vi "ReadWriteTablesTest_1212_K7.vi"() -> ()   [LabVIEW 2018]
uses:
  <vilib>/Platform/TimedLoop/XDataNode/XDataNode.xnode
  <vilib>/Platform/TimedLoop/XDataNode/nitl_modes.ctl
  <vilib>/Platform/TimedLoop/XDataNode/XDNodeRunTimeDep.lvlib
  <vilib>/Platform/TimedLoop/XDataNode/wakeup.ctl
  <vilib>/Platform/TimedLoop/XDataNode/timing_clust.ctl
  <vilib>/rvi/DataTransferAndStorage/Container/XNode/niFpgaContainer.xnode
  <vilib>/eio/EIONode/EIONode.xnode
  <vilib>/rvi/Memory/Memory_Emulation/nirvimemoryEmulation.vi
  <vilib>/rvi/eio/common/nirviEmuTemplateMethod_errors.vi
  <vilib>/rvi/Memory/Memory_Emulation/nirvimemoryFastEmulation.vi
  Program_Files/Labview2018/MAIN/instr.lib/_niInstr/Basic Elements/v1/FPGA/niInstr Basic Elements v1 FPGA.lvlib
  GeneratorStates.ctl
panel:
  out "pulse period":u32
  in  "TrigDigi":bool
  in  "Vi_Trig/nStage_Trig":bool=TRUE
  in  "Trig In":bool
  out "IO Module\\trig_in Edge Detected":bool=TRUE
  in  "Delay bw waves [cycles]":u32
  in  "Waves Per Pixel":i16=1
  out "busy_ni2c":bool
  in  "Trig Selection":bool
  in  "Trig Reset":bool
  in  "Offset_CH1":u32
  in  "Offset_CH0":u32
  in  "START_CH":bool
  in  "Clock SEL":bool
  out "ReadDataI2c":fxp<+,8,8>
  in  "StartRDI2c":bool
  in  "StartWRI2c":bool
  in  "DataI2c5":fxp<+,8,8>
  in  "DataI2c4":fxp<+,8,8>
  in  "DataI2c3":fxp<+,8,8>
  in  "DataI2c2":fxp<+,8,8>
  in  "DataI2c1":fxp<+,8,8>
  in  "DataI2c0":fxp<+,8,8>
  out "START MAST CH1":bool
  out "START MAST CH0":bool
  in  "WRITE MEM CH1":bool
  in  "DDS/ARB CH1":bool=TRUE
  in  "LastAddress_CH1":u32
  in  "Increment_CH1":u32=8
  in  "EN_CH1":bool
  in  "ClkEnable":bool
  in  "WriteAddress":u32
  in  "WriteData":fxp<+,14,14>
  in  "WRITE MEM CH0":bool
  out "Data16":fxp<+,14,14>=8192.0
  in  "StopAddress8_CH1":u32=6143
  out "Data15":fxp<+,14,14>=8192.0
  in  "StopAddress7_CH1":u32=6142
  out "Data14":fxp<+,14,14>=8192.0
  in  "StopAddress6_CH1":u32=6141
  out "Data13":fxp<+,14,14>=8192.0
  in  "StopAddress5_CH1":u32=6140
  out "Data12":fxp<+,14,14>=8192.0
  in  "StopAddress4_CH1":u32=6139
  out "Data11":fxp<+,14,14>=8192.0
  in  "StopAddress3_CH1":u32=6138
  out "Data10":fxp<+,14,14>=8192.0
  in  "StopAddress2_CH1":u32=6137
  out "Data9":fxp<+,14,14>=8192.0
  in  "StopAddress1_CH1":u32=6136
  out "Data8":fxp<+,14,14>=8192.0
  in  "StopAddress8_CH0":u32=6143
  out "Data7":fxp<+,14,14>=8192.0
  in  "StopAddress7_CH0":u32=6142
  out "Data6":fxp<+,14,14>=8192.0
  in  "StopAddress6_CH0":u32=6141
  out "Data5":fxp<+,14,14>=8192.0
  in  "StopAddress5_CH0":u32=6140
  out "Data4":fxp<+,14,14>=8192.0
  in  "StopAddress4_CH0":u32=6139
  out "Data3":fxp<+,14,14>=8192.0
  in  "StopAddress3_CH0":u32=6138
  out "Data1":fxp<+,14,14>=8192.0
  in  "StopAddress1_CH0":u32=6136
  in  "StopAddress2_CH0":u32=6137
  in  "LastAddress_CH0":u32
  out "Data2":fxp<+,14,14>=8192.0
  in  "EN_CH0":bool
  in  "StartAddress7_CH1":u32=6
  in  "StartAddress4_CH1":u32=3
  in  "StartAddress1_CH1":u32
  in  "StartAddress8_CH1":u32=7
  in  "StartAddress6_CH1":u32=5
  in  "StartAddress5_CH1":u32=4
  in  "StartAddress2_CH1":u32=1
  in  "StartAddress3_CH1":u32=2
  in  "StartAddress8_CH0":u32=7
  in  "StartAddress7_CH0":u32=6
  in  "StartAddress6_CH0":u32=5
  in  "StartAddress5_CH0":u32=4
  in  "StartAddress4_CH0":u32=3
  in  "StartAddress3_CH0":u32=2
  in  "StartAddress2_CH0":u32=1
  in  "StartAddress1_CH0":u32
  in  "SysReset":bool
  in  "IO Module\\trig_out":bool
  out "IO Module\\lockedfast":bool
  out "IO Module\\trig_in":bool=TRUE
  in  "DDS/ARB CH0":bool=TRUE
  in  "Increment_CH0":u32=8
  out "error out":errorcluster
  in  "error in (no error)":errorcluster
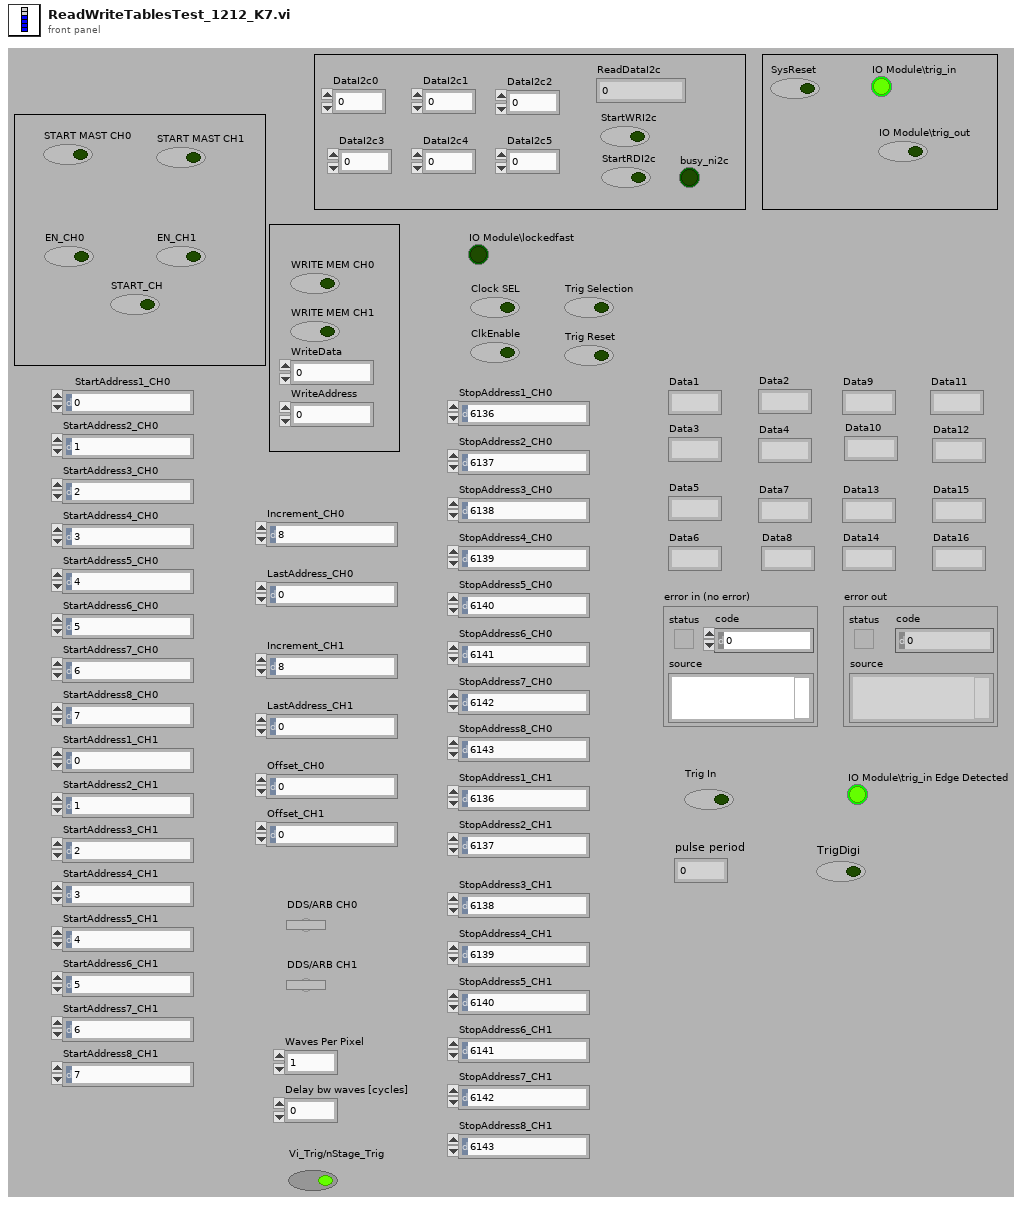
[diagram p1: front panel]
types:
  T1 = typedef "GeneratorStates.ctl" = enum16{"Wait For Trigger", "Wait For Pulse", "Check Pulse Count", "Delay"}
  T2 = typedef "XDNodeRunTimeDep.lvlib/timing_clust.ctl" = cluster{"Expected End [f-1]":u64, "Actual End [f-1]":u64, "Finished Late? [f-1]":bool, "Expected End [i-1]":u64, "Actual End [i-1]":u64, "Finished Late? [i-1]":bool, "Expected Start [i]":u64, "Actual Start [i]":u64, "Expected Start [f]":u64, "Actual Start [f]":u64, "Source Name":string, "Structure Name":string, "Period":i64, "Deadline":i64, "Offset":i64, "Start":i64, "Priority":i32, "Timeout":i32, "Mode":T3, "Wakeup Reason":T4, "Error":errorcluster, "Source Type":string, "Secondary Source Type":string, "Global End Time":u64, "Global Start Time":u64, "Frame Duration":u64, "Iteration Duration":u64, "Assigned CPU":i32, "I/O Scan Engine Mode":u32}
  T3 = typedef "XDNodeRunTimeDep.lvlib/nitl_modes.ctl" = enum32{"No Change", "Process missed periods, maintain original phase", "Discard missed periods, maintain original phase", "Process missed periods, ignore original phase", "Discard missed periods, ignore original phase"}
  T4 = typedef "XDNodeRunTimeDep.lvlib/wakeup.ctl" = enum32{"Normal", "Aborted", "Asynchronous wakeup", "Timing source error", "Timed loop error", "Timeout"}
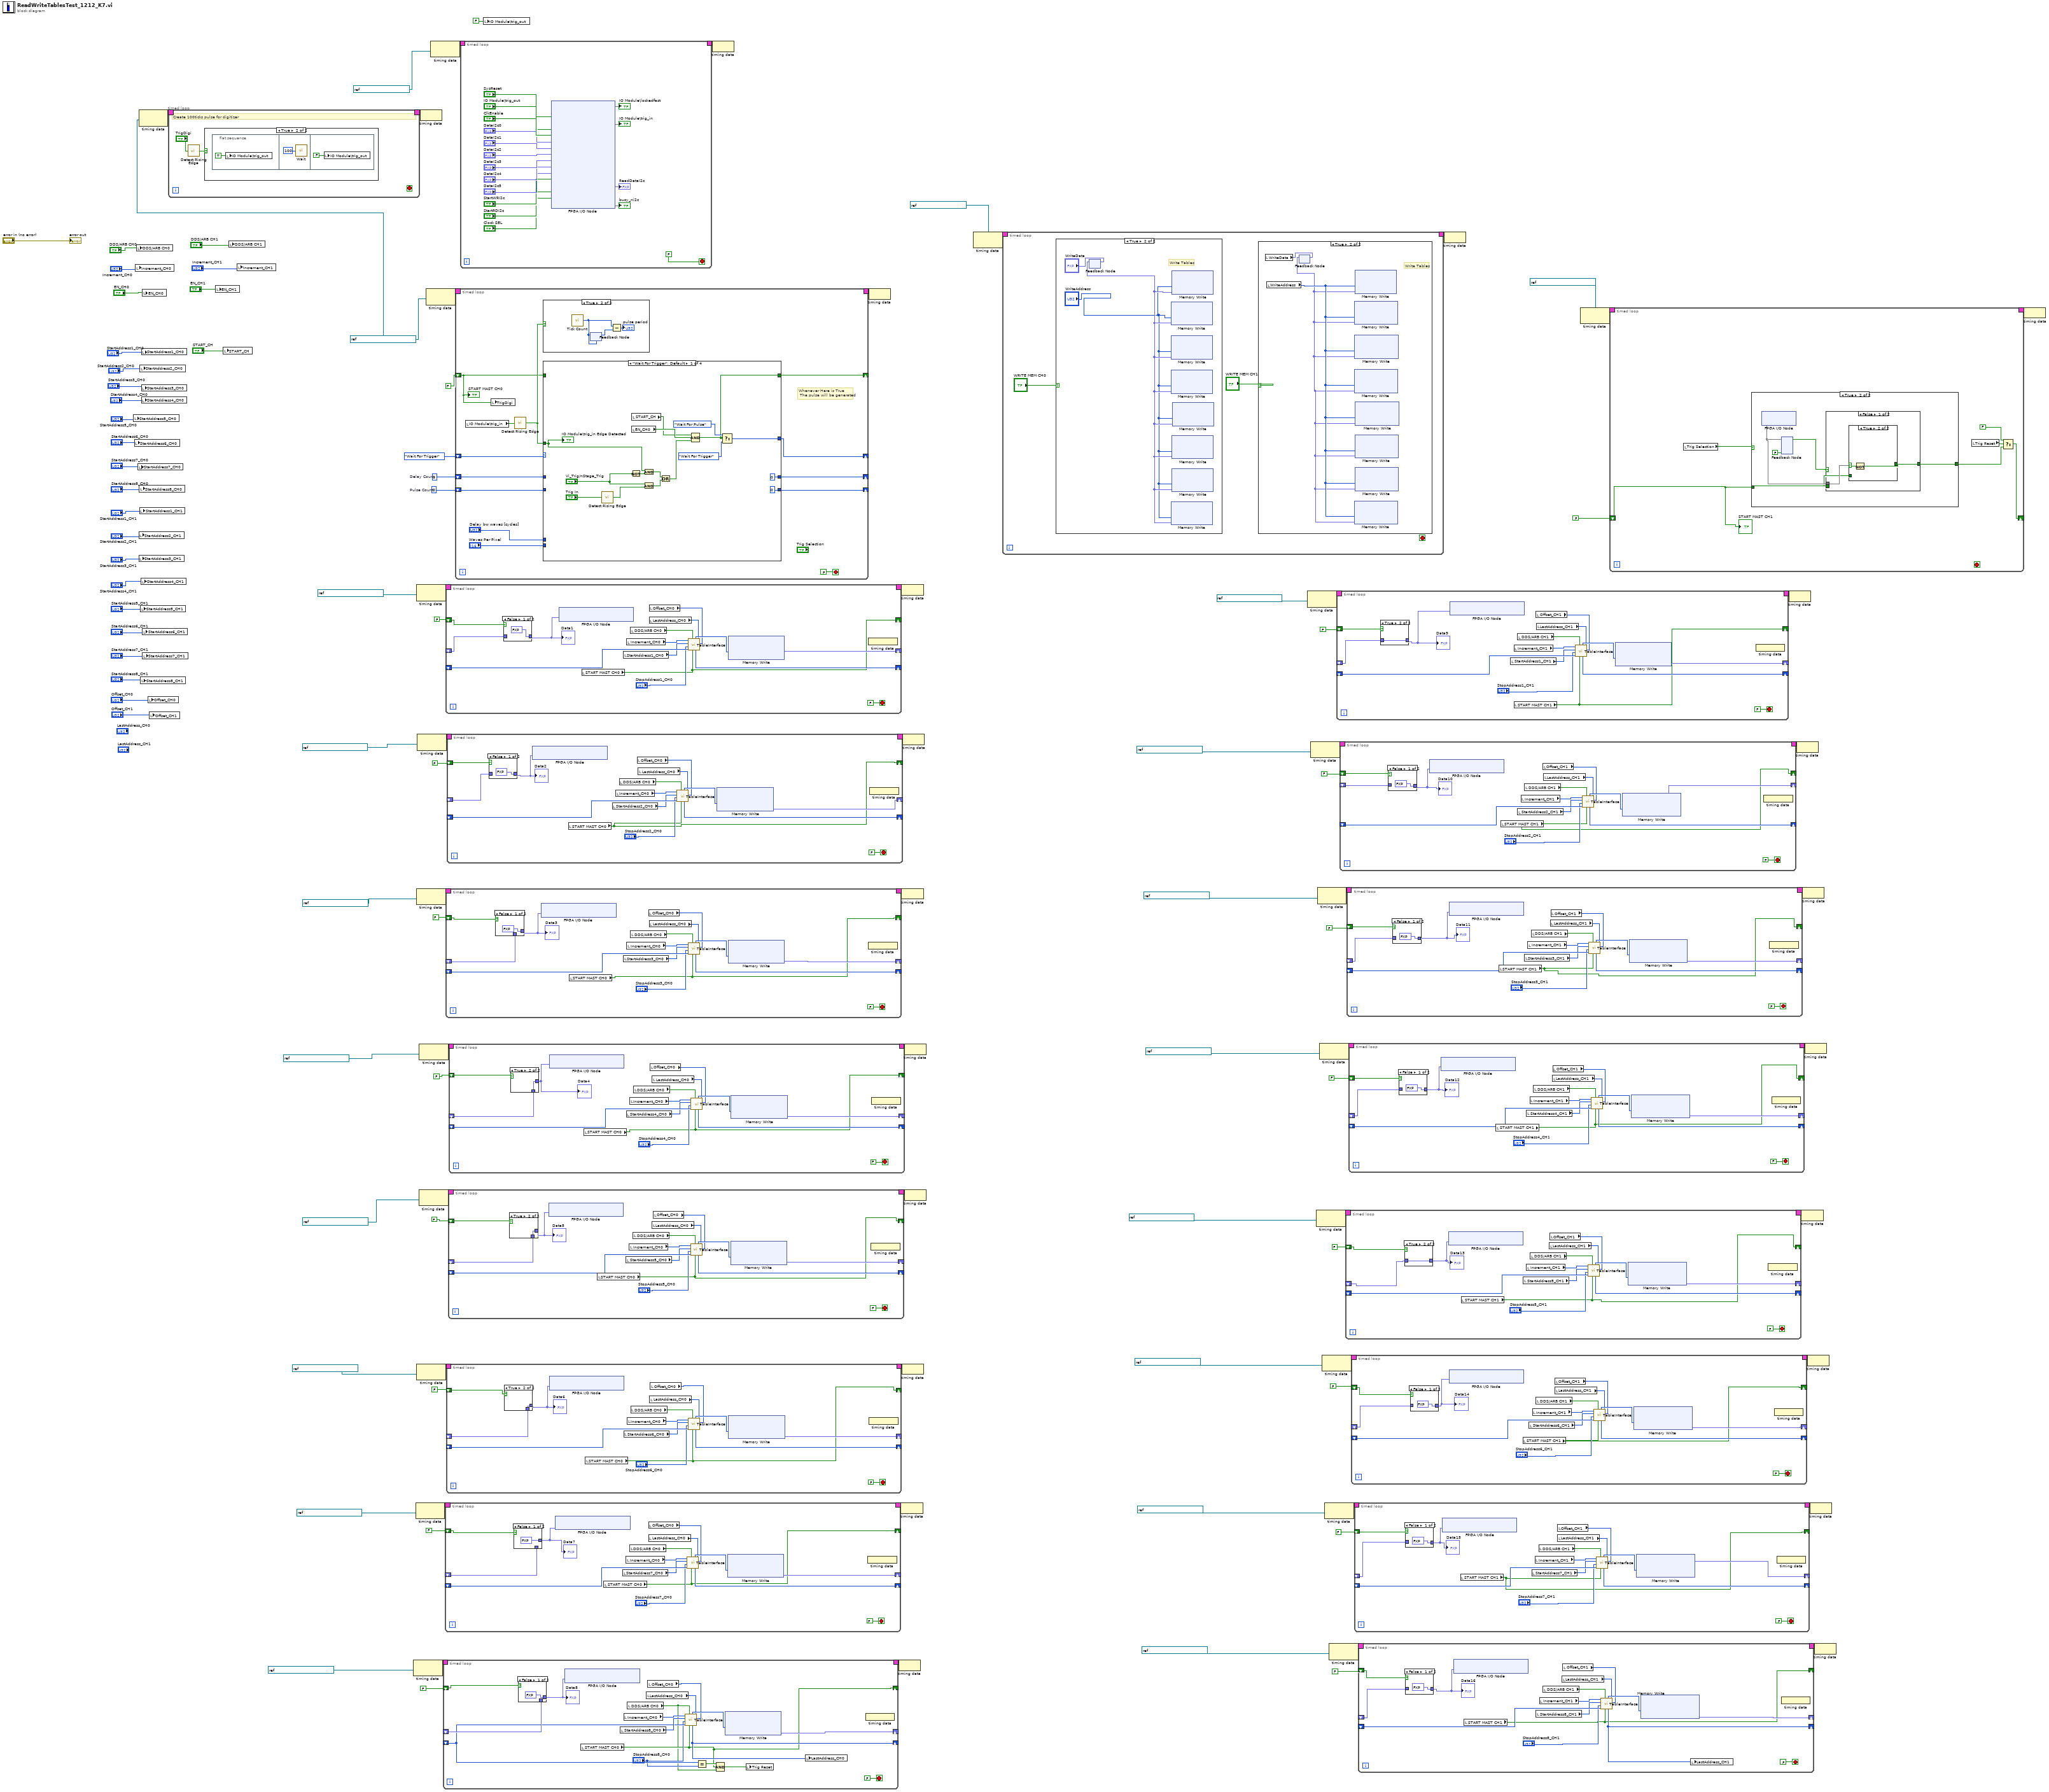
[diagram p0: block diagram]
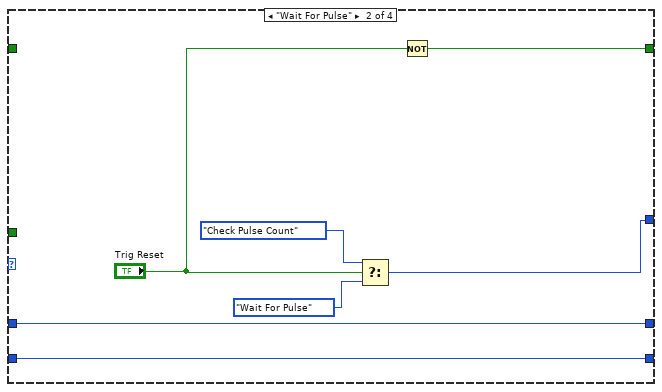
[diagram p4: hidden frame]
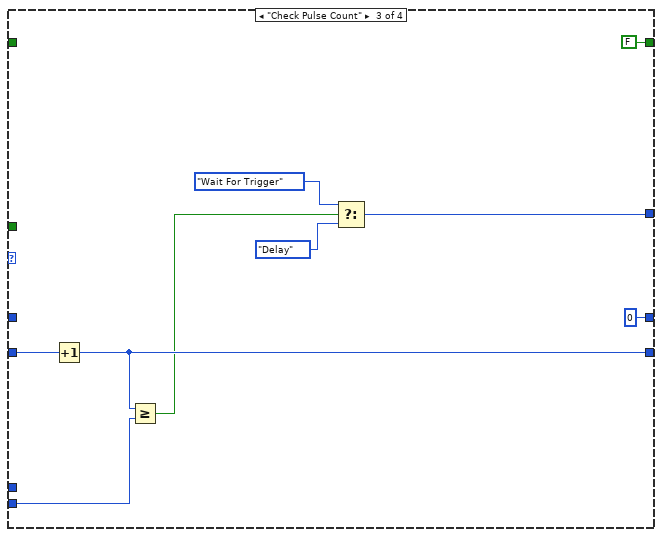
[diagram p5: hidden frame]
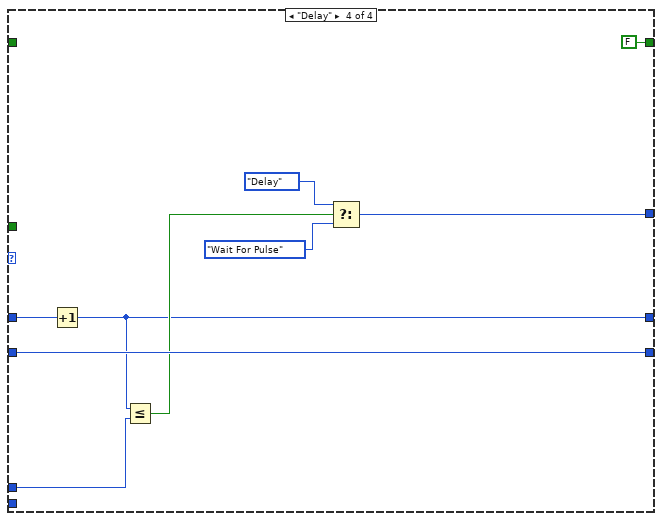
[diagram p6: hidden frame]
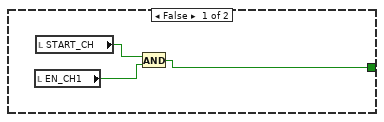
[diagram p7: hidden frame]
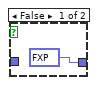
[diagram p15: hidden frame]
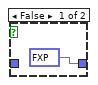
[diagram p19: hidden frame]
diagram:
  w6 = u32 0  # Delay Count
  w7 = i16 0  # Pulse Count
  w2 = refnum<k21> "IO Module\\iomodclipclock0" ("Source Name")
  n1 = local write "StartAddress5_CH0"("StartAddress5_CH0") -> ()
  n2 = local write "StartAddress6_CH0"("StartAddress6_CH0") -> ()
  n3 = local write "Increment_CH0"("Increment_CH0") -> ()
  n4 = local write "DDS/ARB CH0"("DDS/ARB CH0") -> ()
  n5 = local write "StartAddress7_CH0"("StartAddress7_CH0") -> ()
  n6 = node-c288(w2) -> (w4:T2)
  n7 = local write "StartAddress2_CH1"("StartAddress2_CH1") -> ()
  n8 = local write "StartAddress3_CH1"("StartAddress3_CH1") -> ()
  n9 = local write "StartAddress8_CH0"("StartAddress8_CH0") -> ()
  n10 = local write "StartAddress1_CH1"("StartAddress1_CH1") -> ()
  n11 = local write "StartAddress2_CH0"("StartAddress2_CH0") -> ()
  n12 = local write "StartAddress5_CH1"("StartAddress5_CH1") -> ()
  n13 = local write "StartAddress8_CH1"("StartAddress8_CH1") -> ()
  n14 = local write "StartAddress4_CH1"("StartAddress4_CH1") -> ()
  n15 = local write "StartAddress1_CH0"("StartAddress1_CH0") -> ()
  n16 = local write "StartAddress3_CH0"("StartAddress3_CH0") -> ()
  n17 = local write "StartAddress4_CH0"("StartAddress4_CH0") -> ()
  n18 = local write "EN_CH0"("EN_CH0") -> ()
  n19 = local write "StartAddress6_CH1"("StartAddress6_CH1") -> ()
  n20 = local write "StartAddress7_CH1"("StartAddress7_CH1") -> ()
  n21 = local write "Offset_CH0"("Offset_CH0") -> ()
  n22 = local write "Offset_CH1"("Offset_CH1") -> ()
  n23 = timed-loop {
    timing: w4 -> [_]
    timing-out: [_] -> w3
    stop <- _ stop-if-true
    # "Create 100ticks pulse for digitizer"
    n24 = call "Detect Rising Edge.vi"("signal"="TrigDigi") -> ("edge detected"=w111:bool)  [unwired: 14 in]
    n25 = case shown="True" w111 {
      frame False {
      }
      frame True {
        n26 = flat-sequence {
          frame #0 {
            n27 = local write "IO Module\\trig_out"(TRUE ("IO Module\\trig_out")) -> ()
          }
          frame #1 {
            n28 = call "Wait"("Count(Ticks)"=u32 100 ("Count(uSec)")) -> ()  [unwired: 1 out]
          }
          frame #2 {
            n29 = local write "IO Module\\trig_out"(FALSE ("IO Module\\trig_out")) -> ()
          }
        }
      }
    }
  }
  n30 = local write "EN_CH1"("EN_CH1") -> ()
  n31 = local write "START_CH"("START_CH") -> ()
  n32 = local write "DDS/ARB CH1"("DDS/ARB CH1") -> ()
  n33 = local write "Increment_CH1"("Increment_CH1") -> ()
  n34 = node-c288(refnum<k21> "IO Module\\iomodclipclock0" ("Source Name")) -> (w70:T2)
  n35 = node-c288(refnum<k21> "IO Module\\iomodclipclock0" ("Source Name")) -> (w72:T2)
  n36 = node-c288(refnum<k21> "IO Module\\iomodclipclock0" ("Source Name")) -> (w85:T2)
  n37 = node-c288(refnum<k21> "IO Module\\iomodclipclock0" ("Source Name")) -> (w83:T2)
  n38 = node-c288(refnum<k21> "IO Module\\iomodclipclock0" ("Source Name")) -> (w74:T2)
  n39 = node-c288(refnum<k21> "IO Module\\iomodclipclock0" ("Source Name")) -> (w106:T2)
  n40 = node-c288(refnum<k21> "IO Module\\iomodclipclock0" ("Source Name")) -> (w79:T2)
  n41 = node-c288(refnum<k21> "IO Module\\iomodclipclock0" ("Source Name")) -> (w81:T2)
  n42 = node-c288(w3) -> ()
  n43 = node-c288(w2) -> (w10:T2)
  n44 = node-c288(refnum<k21> "40 MHz Onboard Clock" ("Source Name")) -> (w109:T2)
  n45 = timed-loop {
    timing: w70 -> [_]
    timing-out: [_] -> w69
    shift-right: [w134] -> _
    shift-left: _ -> [w123]
    shift-right: [w128] -> _
    shift-left: _ -> [w127]
    shift-right: [w120] -> _
    shift-left: FALSE ("START MAST CH1") -> [w124]
    stop <- FALSE stop-if-true
    n46 = case shown="False" w124 {
      tunnel: [fxp<+,14,14> 8192.0 ("Data2 2") w136] -> w126
      tunnel: w127 -> [_ w136]
      frame False {
      }
      frame True {
      }
    }
    "Data8" <- w126
    n47 = xnode "FPGA I/O Node"("IO Module\\DataDAC_In7_CH0"=w126) -> ()  [unwired: 1 in, 1 out]
    n48 = local read "START MAST CH0"() -> (w120:bool)
    n49 = local read "StartAddress8_CH0"() -> (w132:u32)
    n50 = local read "Increment_CH0"() -> (w133:u32)
    n51 = local read "DDS/ARB CH0"() -> (w119:bool)
    n52 = local read "LastAddress_CH0"() -> (w130:u32)
    n53 = local read "Offset_CH0"() -> (w129:u32)
    n54 = call "TableInterface.vi"("Offset"=w129, "LastAddress"=w130, "START"=w120, "DDS/ARB"=w119, "CurrentAddress"=w123, "StopAddress"="StopAddress8_CH0", "StartAddress"=w132, "Increment"=w133) -> ("NextAddress"=w134:u32, "AddressRam"=w131:u32)  [unwired: 1 in, 1 out]
    n55 = Equal?(x=w123, y="StopAddress8_CH0") -> (x = y?=w121:bool)
    n56 = Compound Arithmetic op=AND(w121, w120, w119) -> (w118:bool)
    n57 = xnode ("Memory Write")("Address"=w131) -> ("Data"=w128:fxp<+,14,14>)  [unwired: 1 in, 1 out]
    n58 = local write "Trig Reset"(w118) -> ()
    n59 = local write "LastAddress_CH0"(w134) -> ()
    n60 = node-c288() -> ()  [unwired: 1 out]
  }
  n61 = timed-loop {
    timing: w72 -> [_]
    timing-out: [_] -> w71
    shift-right: [w153] -> _
    shift-left: _ -> [w152]
    shift-right: [w144] -> _
    shift-left: _ -> [w143]
    shift-right: [w140] -> _
    shift-left: FALSE ("START MAST CH1") -> [w139]
    stop <- FALSE stop-if-true
    n62 = case shown="False" w139 {
      tunnel: w143 -> [_ w155]
      tunnel: [fxp<+,14,14> 8192.0 ("Data2 2") w155] -> w142
      frame False {
      }
      frame True {
      }
    }
    "Data7" <- w142
    n63 = xnode "FPGA I/O Node"("IO Module\\DataDAC_In6_CH0"=w142) -> ()  [unwired: 1 in, 1 out]
    n64 = local read "START MAST CH0"() -> (w140:bool)
    n65 = local read "StartAddress7_CH0"() -> (w150:u32)
    n66 = local read "Increment_CH0"() -> (w151:u32)
    n67 = local read "DDS/ARB CH0"() -> (w148:bool)
    n68 = local read "Offset_CH0"() -> (w145:u32)
    n69 = local read "LastAddress_CH0"() -> (w147:u32)
    n70 = call "TableInterface.vi"("Offset"=w145, "LastAddress"=w147, "START"=w140, "DDS/ARB"=w148, "CurrentAddress"=w152, "StopAddress"="StopAddress7_CH0", "StartAddress"=w150, "Increment"=w151) -> ("NextAddress"=w153:u32, "AddressRam"=w149:u32)  [unwired: 1 in, 1 out]
    n71 = xnode ("Memory Write")("Address"=w149) -> ("Data"=w144:fxp<+,14,14>)  [unwired: 1 in, 1 out]
    n72 = node-c288() -> ()  [unwired: 1 out]
  }
  n73 = timed-loop {
    timing: w85 -> [_]
    timing-out: [_] -> w84
    shift-right: [w172] -> _
    shift-left: _ -> [w171]
    shift-right: [w163] -> _
    shift-left: _ -> [w162]
    shift-right: [w159] -> _
    shift-left: FALSE ("START MAST CH1") -> [w158]
    stop <- FALSE stop-if-true
    n74 = case shown="False" w158 {
      tunnel: [fxp<+,14,14> 8192.0 ("Data2 2") w174] -> w161
      tunnel: w162 -> [_ w174]
      frame False {
      }
      frame True {
      }
    }
    "Data1" <- w161
    n75 = xnode "FPGA I/O Node"("IO Module\\DataDAC_In0_CH0"=w161) -> ()  [unwired: 1 in, 1 out]
    n76 = local read "START MAST CH0"() -> (w159:bool)
    n77 = local read "StartAddress1_CH0"() -> (w169:u32)
    n78 = local read "Increment_CH0"() -> (w170:u32)
    n79 = local read "DDS/ARB CH0"() -> (w167:bool)
    n80 = local read "Offset_CH0"() -> (w164:u32)
    n81 = local read "LastAddress_CH0"() -> (w166:u32)
    n82 = call "TableInterface.vi"("Offset"=w164, "LastAddress"=w166, "START"=w159, "DDS/ARB"=w167, "CurrentAddress"=w171, "StopAddress"="StopAddress1_CH0", "StartAddress"=w169, "Increment"=w170) -> ("NextAddress"=w172:u32, "AddressRam"=w168:u32)  [unwired: 1 in, 1 out]
    n83 = xnode ("Memory Write")("Address"=w168) -> ("Data"=w163:fxp<+,14,14>)  [unwired: 1 in, 1 out]
    n84 = node-c288() -> ()  [unwired: 1 out]
  }
  n85 = timed-loop {
    timing: w83 -> [_]
    timing-out: [_] -> w82
    shift-right: [w191] -> _
    shift-left: _ -> [w190]
    shift-right: [w182] -> _
    shift-left: _ -> [w181]
    shift-right: [w178] -> _
    shift-left: FALSE ("START MAST CH1") -> [w177]
    stop <- FALSE stop-if-true
    n86 = case shown="False" w177 {
      tunnel: [fxp<+,14,14> 8192.0 ("Data2 2") w193] -> w180
      tunnel: w181 -> [_ w193]
      frame False {
      }
      frame True {
      }
    }
    "Data3" <- w180
    n87 = xnode "FPGA I/O Node"("IO Module\\DataDAC_In2_CH0"=w180) -> ()  [unwired: 1 in, 1 out]
    n88 = local read "START MAST CH0"() -> (w178:bool)
    n89 = local read "StartAddress3_CH0"() -> (w188:u32)
    n90 = local read "Increment_CH0"() -> (w189:u32)
    n91 = local read "DDS/ARB CH0"() -> (w186:bool)
    n92 = local read "Offset_CH0"() -> (w183:u32)
    n93 = local read "LastAddress_CH0"() -> (w185:u32)
    n94 = call "TableInterface.vi"("Offset"=w183, "LastAddress"=w185, "START"=w178, "DDS/ARB"=w186, "CurrentAddress"=w190, "StopAddress"="StopAddress3_CH0", "StartAddress"=w188, "Increment"=w189) -> ("NextAddress"=w191:u32, "AddressRam"=w187:u32)  [unwired: 1 in, 1 out]
    n95 = xnode ("Memory Write")("Address"=w187) -> ("Data"=w182:fxp<+,14,14>)  [unwired: 1 in, 1 out]
    n96 = node-c288() -> ()  [unwired: 1 out]
  }
  n97 = timed-loop {
    timing: w74 -> [_]
    timing-out: [_] -> w73
    shift-right: [w210] -> _
    shift-left: _ -> [w209]
    shift-right: [w201] -> _
    shift-left: _ -> [w200]
    shift-right: [w197] -> _
    shift-left: FALSE ("START MAST CH1") -> [w196]
    stop <- FALSE stop-if-true
    n98 = case shown="True" w196 {
      tunnel: [fxp<+,14,14> 8192.0 ("Data2 2") w212] -> w199
      tunnel: w200 -> [_ w212]
      frame False {
      }
      frame True {
      }
    }
    "Data6" <- w199
    n99 = xnode "FPGA I/O Node"("IO Module\\DataDAC_In5_CH0"=w199) -> ()  [unwired: 1 in, 1 out]
    n100 = local read "START MAST CH0"() -> (w197:bool)
    n101 = local read "StartAddress6_CH0"() -> (w207:u32)
    n102 = local read "Increment_CH0"() -> (w208:u32)
    n103 = local read "DDS/ARB CH0"() -> (w205:bool)
    n104 = local read "LastAddress_CH0"() -> (w204:u32)
    n105 = local read "Offset_CH0"() -> (w202:u32)
    n106 = call "TableInterface.vi"("Offset"=w202, "LastAddress"=w204, "START"=w197, "DDS/ARB"=w205, "CurrentAddress"=w209, "StopAddress"="StopAddress6_CH0", "StartAddress"=w207, "Increment"=w208) -> ("NextAddress"=w210:u32, "AddressRam"=w206:u32)  [unwired: 1 in, 1 out]
    n107 = xnode ("Memory Write")("Address"=w206) -> ("Data"=w201:fxp<+,14,14>)  [unwired: 1 in, 1 out]
    n108 = node-c288() -> ()  [unwired: 1 out]
  }
  n109 = timed-loop {
    timing: w106 -> [_]
    timing-out: [_] -> w105
    shift-right: [w229] -> _
    shift-left: _ -> [w228]
    shift-right: [w220] -> _
    shift-left: _ -> [w219]
    shift-right: [w216] -> _
    shift-left: FALSE ("START MAST CH1") -> [w215]
    stop <- FALSE stop-if-true
    n110 = case shown="False" w215 {
      tunnel: [fxp<+,14,14> 8192.0 ("Data2 2") w231] -> w218
      tunnel: w219 -> [_ w231]
      frame False {
      }
      frame True {
      }
    }
    "Data2" <- w218
    n111 = xnode "FPGA I/O Node"("IO Module\\DataDAC_In1_CH0"=w218) -> ()  [unwired: 1 in, 1 out]
    n112 = local read "START MAST CH0"() -> (w216:bool)
    n113 = local read "StartAddress2_CH0"() -> (w226:u32)
    n114 = local read "Increment_CH0"() -> (w227:u32)
    n115 = local read "DDS/ARB CH0"() -> (w224:bool)
    n116 = local read "Offset_CH0"() -> (w221:u32)
    n117 = local read "LastAddress_CH0"() -> (w223:u32)
    n118 = call "TableInterface.vi"("Offset"=w221, "LastAddress"=w223, "START"=w216, "DDS/ARB"=w224, "CurrentAddress"=w228, "StopAddress"="StopAddress2_CH0", "StartAddress"=w226, "Increment"=w227) -> ("NextAddress"=w229:u32, "AddressRam"=w225:u32)  [unwired: 1 in, 1 out]
    n119 = xnode ("Memory Write")("Address"=w225) -> ("Data"=w220:fxp<+,14,14>)  [unwired: 1 in, 1 out]
    n120 = node-c288() -> ()  [unwired: 1 out]
  }
  n121 = timed-loop {
    timing: w79 -> [_]
    timing-out: [_] -> w78
    shift-right: [w248] -> _
    shift-left: _ -> [w247]
    shift-right: [w239] -> _
    shift-left: _ -> [w238]
    shift-right: [w235] -> _
    shift-left: FALSE ("START MAST CH1") -> [w234]
    stop <- FALSE stop-if-true
    n122 = case shown="True" w234 {
      tunnel: [fxp<+,14,14> 8192.0 ("Data2 2") w250] -> w237
      tunnel: w238 -> [_ w250]
      frame False {
      }
      frame True {
      }
    }
    "Data5" <- w237
    n123 = xnode "FPGA I/O Node"("IO Module\\DataDAC_In4_CH0"=w237) -> ()  [unwired: 1 in, 1 out]
    n124 = local read "START MAST CH0"() -> (w235:bool)
    n125 = local read "StartAddress5_CH0"() -> (w245:u32)
    n126 = local read "Increment_CH0"() -> (w246:u32)
    n127 = local read "DDS/ARB CH0"() -> (w243:bool)
    n128 = local read "LastAddress_CH0"() -> (w242:u32)
    n129 = local read "Offset_CH0"() -> (w240:u32)
    n130 = call "TableInterface.vi"("Offset"=w240, "LastAddress"=w242, "START"=w235, "DDS/ARB"=w243, "CurrentAddress"=w247, "StopAddress"="StopAddress5_CH0", "StartAddress"=w245, "Increment"=w246) -> ("NextAddress"=w248:u32, "AddressRam"=w244:u32)  [unwired: 1 in, 1 out]
    n131 = xnode ("Memory Write")("Address"=w244) -> ("Data"=w239:fxp<+,14,14>)  [unwired: 1 in, 1 out]
    n132 = node-c288() -> ()  [unwired: 1 out]
  }
  n133 = timed-loop {
    timing: w81 -> [_]
    timing-out: [_] -> w80
    shift-right: [w267] -> _
    shift-left: _ -> [w266]
    shift-right: [w258] -> _
    shift-left: _ -> [w257]
    shift-right: [w254] -> _
    shift-left: FALSE ("START MAST CH1") -> [w253]
    stop <- FALSE stop-if-true
    n134 = case shown="True" w253 {
      tunnel: [fxp<+,14,14> 8192.0 ("Data2 2") w269] -> w256
      tunnel: w257 -> [_ w269]
      frame False {
      }
      frame True {
      }
    }
    "Data4" <- w256
    n135 = xnode "FPGA I/O Node"("IO Module\\DataDAC_In3_CH0"=w256) -> ()  [unwired: 1 in, 1 out]
    n136 = local read "START MAST CH0"() -> (w254:bool)
    n137 = local read "StartAddress4_CH0"() -> (w264:u32)
    n138 = local read "Increment_CH0"() -> (w265:u32)
    n139 = local read "DDS/ARB CH0"() -> (w262:bool)
    n140 = local read "Offset_CH0"() -> (w259:u32)
    n141 = local read "LastAddress_CH0"() -> (w261:u32)
    n142 = call "TableInterface.vi"("Offset"=w259, "LastAddress"=w261, "START"=w254, "DDS/ARB"=w262, "CurrentAddress"=w266, "StopAddress"="StopAddress4_CH0", "StartAddress"=w264, "Increment"=w265) -> ("NextAddress"=w267:u32, "AddressRam"=w263:u32)  [unwired: 1 in, 1 out]
    n143 = xnode ("Memory Write")("Address"=w263) -> ("Data"=w258:fxp<+,14,14>)  [unwired: 1 in, 1 out]
    n144 = node-c288() -> ()  [unwired: 1 out]
  }
  n145 = timed-loop {
    timing: w10 -> [_]
    timing-out: [_] -> w9
    shift-right: [w273] -> _
    shift-left: FALSE -> [w272]
    shift-right: [w283] -> _
    shift-left: w7 -> [w278]
    shift-right: [w281] -> _
    shift-left: w6 -> [w282]
    shift-right: [w276] -> _
    shift-left: GeneratorStates."Wait For Trigger" -> [w277]
    stop <- FALSE stop-if-true
    # "Whenever Here is True\n The pulse will be generated"
    n146 = local read "IO Module\\trig_in"() -> (w275:bool)
    n147 = local write "TrigDigi"(w272) -> ()
    n148 = call "Detect Rising Edge.vi"("signal"=w275) -> ("edge detected"=w274:bool)  [unwired: 14 in]
    n149 = case shown="\"Wait For Trigger\", Default" w277 {
      tunnel: [w289 w307 FALSE FALSE] -> w273
      tunnel: w272 -> [_ _ _ _]
      tunnel: w278 -> [_ w309 w319 w328]
      tunnel: [i16 0 ("Pulse Count") w309 w318 w328] -> w283
      tunnel: w282 -> [_ w308 _ w327]
      tunnel: [i16 0 ("Delay Count") w308 u32 0 ("Delay Count") w323] -> w281
      tunnel: "Delay bw waves [cycles]" -> [_ _ _ w322]
      tunnel: "Waves Per Pixel" -> [_ _ w317 _]
      tunnel: [w292 w305 w311 w320] -> w276
      tunnel: w274 -> [w288 _ _ _]
      frame "Wait For Trigger", Default {
        n150 = call "Detect Rising Edge.vi"("signal"="Trig In") -> ("edge detected"=w302:bool)  [unwired: 14 in]
        n151 = Not(x="Vi_Trig/nStage_Trig") -> (.not. x?=w297:bool)
        n152 = local read "EN_CH0"() -> (w291:bool)
        n153 = local read "START_CH"() -> (w290:bool)
        n154 = And(x=w288, y=w297) -> (x .and. y?=w300:bool)
        n155 = And(x="Vi_Trig/nStage_Trig", y=w302) -> (x .and. y?=w299:bool)
        n156 = Or(x=w300, y=w299) -> (x .or. y?=w301:bool)
        n157 = Compound Arithmetic op=AND(w290, w291, w301) -> (w289:bool)
        n158 = Select(t=GeneratorStates."Wait For Pulse", s=w289, f=GeneratorStates."Wait For Trigger") -> (s? t:f=w292:T1)
        "IO Module\\trig_in Edge Detected" <- w288
      }
      frame "Wait For Pulse" {
        n159 = Select(t=GeneratorStates."Check Pulse Count", s="Trig Reset", f=GeneratorStates."Wait For Pulse") -> (s? t:f=w305:T1)
        n160 = Not(x="Trig Reset") -> (.not. x?=w307:bool)
      }
      frame "Check Pulse Count" {
        n161 = Increment(x=w319) -> (x+1=w318:i16)
        n162 = Greater Or Equal?(x=w318, y=w317) -> (x >= y?=w314:bool)
        n163 = Select(t=GeneratorStates."Wait For Trigger", s=w314, f=GeneratorStates."Delay") -> (s? t:f=w311:T1)
      }
      frame "Delay" {
        n164 = Increment(x=w327) -> (x+1=w323:u32)
        n165 = Less Or Equal?(x=w323, y=w322) -> (x <= y?=w324:bool)
        n166 = Select(t=GeneratorStates."Delay", s=w324, f=GeneratorStates."Wait For Pulse") -> (s? t:f=w320:T1)
      }
    }
    n167 = case shown="True" w274 {
      frame False {
      }
      frame True {
        n168 = call "Tick Count"() -> ("Tick Count(Ticks)"=w286:u32)
        n169 = feedback #1(w286) -> (w287:u32)
        n170 = feedback-in #1(w286) -> ()
        n171 = Subtract(x=w286, y=w287) -> (x-y=→"pulse period":u32)
      }
    }
    "START MAST CH0" <- w272
  }
  n172 = timed-loop {
    timing: w109 -> [_]
    timing-out: [_] -> w108
    stop <- FALSE stop-if-true
    n173 = xnode "FPGA I/O Node"("IO Module\\reset_in"="SysReset", "IO Module\\Trig_out"="IO Module\\trig_out", "IO Module\\ClkEnable"="ClkEnable", "IO Module\\DataI2C0"="DataI2c0", "IO Module\\DataI2C1"="DataI2c1", "IO Module\\DataI2C2"="DataI2c2", "IO Module\\DataI2C3"="DataI2c3", "IO Module\\DataI2C4"="DataI2c4", "IO Module\\DataI2C5"="DataI2c5", "IO Module\\StartWRI2C"="StartWRI2c", "IO Module\\StartRDI2C"="StartRDI2c", "IO Module\\ClockSel"="Clock SEL") -> ("IO Module\\LockedFast"=→"IO Module\\lockedfast", "IO Module\\Trig_in"=→"IO Module\\trig_in", "IO Module\\ReadDataI2C"=→"ReadDataI2c", "IO Module\\Busy_nI2C"=→"busy_ni2c")  [unwired: 16 in, 16 out]
  }
  n174 = local write "IO Module\\trig_out"(FALSE ("IO Module\\trig_out")) -> ()
  n175 = node-c288(w108) -> ()
  n176 = node-c288(w9) -> ()
  n177 = node-c288(w69) -> ()
  n178 = node-c288(w71) -> ()
  n179 = node-c288(w84) -> ()
  n180 = node-c288(w82) -> ()
  n181 = node-c288(w73) -> ()
  n182 = node-c288(w105) -> ()
  n183 = node-c288(w78) -> ()
  n184 = node-c288(w80) -> ()
  n185 = node-c288(refnum<k21> "40 MHz Onboard Clock" ("Source Name")) -> (w40:T2)
  n186 = timed-loop {
    timing: w40 -> [_]
    timing-out: [_] -> w39
    stop <- _ stop-if-true
    n187 = case shown="True" "WRITE MEM CH0" {
      frame False {
      }
      frame True {
        # "Write Tables"
        n188 = feedback #2() -> (w356:fxp<+,14,14>)  [unwired: 1 in]
        n189 = feedback-in #2("WriteData") -> ()
        n190 = xnode ("Memory Write")("Address"="WriteAddress", "Data"=w356) -> ()  [unwired: 1 in, 1 out]
        n191 = xnode ("Memory Write")("Address"="WriteAddress", "Data"=w356) -> ()  [unwired: 1 in, 1 out]
        n192 = xnode ("Memory Write")("Address"="WriteAddress", "Data"=w356) -> ()  [unwired: 1 in, 1 out]
        n193 = xnode ("Memory Write")("Address"="WriteAddress", "Data"=w356) -> ()  [unwired: 1 in, 1 out]
        n194 = xnode ("Memory Write")("Address"="WriteAddress", "Data"=w356) -> ()  [unwired: 1 in, 1 out]
        n195 = xnode ("Memory Write")("Address"="WriteAddress", "Data"=w356) -> ()  [unwired: 1 in, 1 out]
        n196 = xnode ("Memory Write")("Address"="WriteAddress", "Data"=w356) -> ()  [unwired: 1 in, 1 out]
        n197 = xnode ("Memory Write")("Address"="WriteAddress", "Data"=w356) -> ()  [unwired: 1 in, 1 out]
      }
    }
    n198 = case shown="True" "WRITE MEM CH1" {
      frame False {
      }
      frame True {
        # "Write Tables"
        n199 = local read "WriteData"() -> (w353:fxp<+,14,14>)
        n200 = local read "WriteAddress"() -> (w354:u32)
        n201 = feedback #3() -> (w352:fxp<+,14,14>)  [unwired: 1 in]
        n202 = feedback-in #3(w353) -> ()
        n203 = xnode ("Memory Write")("Address"=w354, "Data"=w352) -> ()  [unwired: 1 in, 1 out]
        n204 = xnode ("Memory Write")("Address"=w354, "Data"=w352) -> ()  [unwired: 1 in, 1 out]
        n205 = xnode ("Memory Write")("Address"=w354, "Data"=w352) -> ()  [unwired: 1 in, 1 out]
        n206 = xnode ("Memory Write")("Address"=w354, "Data"=w352) -> ()  [unwired: 1 in, 1 out]
        n207 = xnode ("Memory Write")("Address"=w354, "Data"=w352) -> ()  [unwired: 1 in, 1 out]
        n208 = xnode ("Memory Write")("Address"=w354, "Data"=w352) -> ()  [unwired: 1 in, 1 out]
        n209 = xnode ("Memory Write")("Address"=w354, "Data"=w352) -> ()  [unwired: 1 in, 1 out]
        n210 = xnode ("Memory Write")("Address"=w354, "Data"=w352) -> ()  [unwired: 1 in, 1 out]
      }
    }
  }
  n211 = node-c288(refnum<k21> "IO Module\\iomodclipclock0" ("Source Name")) -> (w68:T2)
  n212 = node-c288(refnum<k21> "IO Module\\iomodclipclock0" ("Source Name")) -> (w61:T2)
  n213 = node-c288(refnum<k21> "IO Module\\iomodclipclock0" ("Source Name")) -> (w52:T2)
  n214 = node-c288(refnum<k21> "IO Module\\iomodclipclock0" ("Source Name")) -> (w58:T2)
  n215 = node-c288(refnum<k21> "IO Module\\iomodclipclock0" ("Source Name")) -> (w55:T2)
  n216 = node-c288(refnum<k21> "IO Module\\iomodclipclock0" ("Source Name")) -> (w49:T2)
  n217 = node-c288(refnum<k21> "IO Module\\iomodclipclock0" ("Source Name")) -> (w46:T2)
  n218 = node-c288(refnum<k21> "IO Module\\iomodclipclock0" ("Source Name")) -> (w43:T2)
  n219 = timed-loop {
    timing: w68 -> [_]
    timing-out: [_] -> w67
    shift-right: [w366] -> _
    shift-left: _ -> [w374]
    shift-right: [w365] -> _
    shift-left: _ -> [w364]
    shift-right: [w361] -> _
    shift-left: FALSE ("START MAST CH2") -> [w360]
    stop <- FALSE stop-if-true
    n220 = case shown="True" w360 {
      tunnel: [fxp<+,14,14> 8192.0 ("Data2 2") w376] -> w363
      tunnel: w364 -> [_ w376]
      frame False {
      }
      frame True {
      }
    }
    "Data9" <- w363
    n221 = xnode "FPGA I/O Node"("IO Module\\DataDAC_In0_CH1"=w363) -> ()  [unwired: 1 in, 1 out]
    n222 = local read "StartAddress1_CH1"() -> (w372:u32)
    n223 = local read "Increment_CH1"() -> (w373:u32)
    n224 = local read "START MAST CH1"() -> (w361:bool)
    n225 = local read "DDS/ARB CH1"() -> (w370:bool)
    n226 = local read "Offset_CH1"() -> (w367:u32)
    n227 = local read "LastAddress_CH1"() -> (w369:u32)
    n228 = call "TableInterface.vi"("Offset"=w367, "LastAddress"=w369, "START"=w361, "DDS/ARB"=w370, "CurrentAddress"=w374, "StopAddress"="StopAddress1_CH1", "StartAddress"=w372, "Increment"=w373) -> ("NextAddress"=w366:u32, "AddressRam"=w371:u32)  [unwired: 1 in, 1 out]
    n229 = xnode ("Memory Write")("Address"=w371) -> ("Data"=w365:fxp<+,14,14>)  [unwired: 1 in, 1 out]
    n230 = node-c288() -> ()  [unwired: 1 out]
  }
  n231 = timed-loop {
    timing: w61 -> [_]
    timing-out: [_] -> w60
    shift-right: [w393] -> _
    shift-left: _ -> [w392]
    shift-right: [w384] -> _
    shift-left: _ -> [w383]
    shift-right: [w380] -> _
    shift-left: FALSE ("START MAST CH2") -> [w379]
    stop <- FALSE stop-if-true
    n232 = case shown="False" w379 {
      tunnel: [fxp<+,14,14> 8192.0 ("Data2 2") w395] -> w382
      tunnel: w383 -> [_ w395]
      frame False {
      }
      frame True {
      }
    }
    "Data10" <- w382
    n233 = xnode "FPGA I/O Node"("IO Module\\DataDAC_In1_CH1"=w382) -> ()  [unwired: 1 in, 1 out]
    n234 = local read "START MAST CH1"() -> (w380:bool)
    n235 = local read "StartAddress2_CH1"() -> (w390:u32)
    n236 = local read "Increment_CH1"() -> (w391:u32)
    n237 = local read "DDS/ARB CH1"() -> (w388:bool)
    n238 = local read "Offset_CH1"() -> (w385:u32)
    n239 = local read "LastAddress_CH1"() -> (w387:u32)
    n240 = call "TableInterface.vi"("Offset"=w385, "LastAddress"=w387, "START"=w380, "DDS/ARB"=w388, "CurrentAddress"=w392, "StopAddress"="StopAddress2_CH1", "StartAddress"=w390, "Increment"=w391) -> ("NextAddress"=w393:u32, "AddressRam"=w389:u32)  [unwired: 1 in, 1 out]
    n241 = xnode ("Memory Write")("Address"=w389) -> ("Data"=w384:fxp<+,14,14>)  [unwired: 1 in, 1 out]
    n242 = node-c288() -> ()  [unwired: 1 out]
  }
  n243 = timed-loop {
    timing: w52 -> [_]
    timing-out: [_] -> w51
    shift-right: [w412] -> _
    shift-left: _ -> [w411]
    shift-right: [w403] -> _
    shift-left: _ -> [w402]
    shift-right: [w399] -> _
    shift-left: FALSE ("START MAST CH2") -> [w398]
    stop <- FALSE stop-if-true
    n244 = case shown="True" w398 {
      tunnel: [fxp<+,14,14> 8192.0 ("Data2 2") w414] -> w401
      tunnel: w402 -> [_ w414]
      frame False {
      }
      frame True {
      }
    }
    "Data13" <- w401
    n245 = xnode "FPGA I/O Node"("IO Module\\DataDAC_In4_CH1"=w401) -> ()  [unwired: 1 in, 1 out]
    n246 = local read "START MAST CH1"() -> (w399:bool)
    n247 = local read "StartAddress5_CH1"() -> (w409:u32)
    n248 = local read "Increment_CH1"() -> (w410:u32)
    n249 = local read "DDS/ARB CH1"() -> (w407:bool)
    n250 = local read "LastAddress_CH1"() -> (w406:u32)
    n251 = local read "Offset_CH1"() -> (w404:u32)
    n252 = call "TableInterface.vi"("Offset"=w404, "LastAddress"=w406, "START"=w399, "DDS/ARB"=w407, "CurrentAddress"=w411, "StopAddress"="StopAddress5_CH1", "StartAddress"=w409, "Increment"=w410) -> ("NextAddress"=w412:u32, "AddressRam"=w408:u32)  [unwired: 1 in, 1 out]
    n253 = xnode ("Memory Write")("Address"=w408) -> ("Data"=w403:fxp<+,14,14>)  [unwired: 1 in, 1 out]
    n254 = node-c288() -> ()  [unwired: 1 out]
  }
  n255 = timed-loop {
    timing: w58 -> [_]
    timing-out: [_] -> w57
    shift-right: [w431] -> _
    shift-left: _ -> [w430]
    shift-right: [w422] -> _
    shift-left: _ -> [w421]
    shift-right: [w418] -> _
    shift-left: FALSE ("START MAST CH2") -> [w417]
    stop <- FALSE stop-if-true
    n256 = case shown="False" w417 {
      tunnel: [fxp<+,14,14> 8192.0 ("Data2 2") w433] -> w420
      tunnel: w421 -> [_ w433]
      frame False {
      }
      frame True {
      }
    }
    "Data11" <- w420
    n257 = xnode "FPGA I/O Node"("IO Module\\DataDAC_In2_CH1"=w420) -> ()  [unwired: 1 in, 1 out]
    n258 = local read "START MAST CH1"() -> (w418:bool)
    n259 = local read "StartAddress3_CH1"() -> (w428:u32)
    n260 = local read "Increment_CH1"() -> (w429:u32)
    n261 = local read "DDS/ARB CH1"() -> (w426:bool)
    n262 = local read "LastAddress_CH1"() -> (w425:u32)
    n263 = local read "Offset_CH1"() -> (w423:u32)
    n264 = call "TableInterface.vi"("Offset"=w423, "LastAddress"=w425, "START"=w418, "DDS/ARB"=w426, "CurrentAddress"=w430, "StopAddress"="StopAddress3_CH1", "StartAddress"=w428, "Increment"=w429) -> ("NextAddress"=w431:u32, "AddressRam"=w427:u32)  [unwired: 1 in, 1 out]
    n265 = xnode ("Memory Write")("Address"=w427) -> ("Data"=w422:fxp<+,14,14>)  [unwired: 1 in, 1 out]
    n266 = node-c288() -> ()  [unwired: 1 out]
  }
  n267 = timed-loop {
    timing: w55 -> [_]
    timing-out: [_] -> w54
    shift-right: [w450] -> _
    shift-left: _ -> [w449]
    shift-right: [w441] -> _
    shift-left: _ -> [w440]
    shift-right: [w437] -> _
    shift-left: FALSE ("START MAST CH2") -> [w436]
    stop <- FALSE stop-if-true
    n268 = case shown="False" w436 {
      tunnel: [fxp<+,14,14> 8192.0 ("Data2 2") w452] -> w439
      tunnel: w440 -> [_ w452]
      frame False {
      }
      frame True {
      }
    }
    "Data12" <- w439
    n269 = xnode "FPGA I/O Node"("IO Module\\DataDAC_In3_CH1"=w439) -> ()  [unwired: 1 in, 1 out]
    n270 = local read "START MAST CH1"() -> (w437:bool)
    n271 = local read "StartAddress4_CH1"() -> (w447:u32)
    n272 = local read "Increment_CH1"() -> (w448:u32)
    n273 = local read "DDS/ARB CH1"() -> (w445:bool)
    n274 = local read "LastAddress_CH1"() -> (w444:u32)
    n275 = local read "Offset_CH1"() -> (w442:u32)
    n276 = call "TableInterface.vi"("Offset"=w442, "LastAddress"=w444, "START"=w437, "DDS/ARB"=w445, "CurrentAddress"=w449, "StopAddress"="StopAddress4_CH1", "StartAddress"=w447, "Increment"=w448) -> ("NextAddress"=w450:u32, "AddressRam"=w446:u32)  [unwired: 1 in, 1 out]
    n277 = xnode ("Memory Write")("Address"=w446) -> ("Data"=w441:fxp<+,14,14>)  [unwired: 1 in, 1 out]
    n278 = node-c288() -> ()  [unwired: 1 out]
  }
  n279 = timed-loop {
    timing: w49 -> [_]
    timing-out: [_] -> w48
    shift-right: [w469] -> _
    shift-left: _ -> [w468]
    shift-right: [w460] -> _
    shift-left: _ -> [w459]
    shift-right: [w456] -> _
    shift-left: FALSE ("START MAST CH2") -> [w455]
    stop <- FALSE stop-if-true
    n280 = case shown="False" w455 {
      tunnel: [fxp<+,14,14> 8192.0 ("Data2 2") w471] -> w458
      tunnel: w459 -> [_ w471]
      frame False {
      }
      frame True {
      }
    }
    "Data14" <- w458
    n281 = xnode "FPGA I/O Node"("IO Module\\DataDAC_In5_CH1"=w458) -> ()  [unwired: 1 in, 1 out]
    n282 = local read "START MAST CH1"() -> (w456:bool)
    n283 = local read "StartAddress6_CH1"() -> (w466:u32)
    n284 = local read "Increment_CH1"() -> (w467:u32)
    n285 = local read "DDS/ARB CH1"() -> (w464:bool)
    n286 = local read "Offset_CH1"() -> (w461:u32)
    n287 = local read "LastAddress_CH1"() -> (w463:u32)
    n288 = call "TableInterface.vi"("Offset"=w461, "LastAddress"=w463, "START"=w456, "DDS/ARB"=w464, "CurrentAddress"=w468, "StopAddress"="StopAddress6_CH1", "StartAddress"=w466, "Increment"=w467) -> ("NextAddress"=w469:u32, "AddressRam"=w465:u32)  [unwired: 1 in, 1 out]
    n289 = xnode ("Memory Write")("Address"=w465) -> ("Data"=w460:fxp<+,14,14>)  [unwired: 1 in, 1 out]
    n290 = node-c288() -> ()  [unwired: 1 out]
  }
  n291 = timed-loop {
    timing: w46 -> [_]
    timing-out: [_] -> w45
    shift-right: [w488] -> _
    shift-left: _ -> [w487]
    shift-right: [w479] -> _
    shift-left: _ -> [w478]
    shift-right: [w475] -> _
    shift-left: FALSE ("START MAST CH2") -> [w474]
    stop <- FALSE stop-if-true
    n292 = case shown="False" w474 {
      tunnel: [fxp<+,14,14> 8192.0 ("Data2 2") w490] -> w477
      tunnel: w478 -> [_ w490]
      frame False {
      }
      frame True {
      }
    }
    "Data15" <- w477
    n293 = xnode "FPGA I/O Node"("IO Module\\DataDAC_In6_CH1"=w477) -> ()  [unwired: 1 in, 1 out]
    n294 = local read "START MAST CH1"() -> (w475:bool)
    n295 = local read "StartAddress7_CH1"() -> (w485:u32)
    n296 = local read "Increment_CH1"() -> (w486:u32)
    n297 = local read "DDS/ARB CH1"() -> (w483:bool)
    n298 = local read "Offset_CH1"() -> (w480:u32)
    n299 = local read "LastAddress_CH1"() -> (w482:u32)
    n300 = call "TableInterface.vi"("Offset"=w480, "LastAddress"=w482, "START"=w475, "DDS/ARB"=w483, "CurrentAddress"=w487, "StopAddress"="StopAddress7_CH1", "StartAddress"=w485, "Increment"=w486) -> ("NextAddress"=w488:u32, "AddressRam"=w484:u32)  [unwired: 1 in, 1 out]
    n301 = xnode ("Memory Write")("Address"=w484) -> ("Data"=w479:fxp<+,14,14>)  [unwired: 1 in, 1 out]
    n302 = node-c288() -> ()  [unwired: 1 out]
  }
  n303 = timed-loop {
    timing: w43 -> [_]
    timing-out: [_] -> w42
    shift-right: [w506] -> _
    shift-left: _ -> [w507]
    shift-right: [w498] -> _
    shift-left: _ -> [w497]
    shift-right: [w494] -> _
    shift-left: FALSE ("START MAST CH2") -> [w493]
    stop <- FALSE stop-if-true
    n304 = case shown="False" w493 {
      tunnel: [fxp<+,14,14> 8192.0 ("Data2 2") w509] -> w496
      tunnel: w497 -> [_ w509]
      frame False {
      }
      frame True {
      }
    }
    "Data16" <- w496
    n305 = xnode "FPGA I/O Node"("IO Module\\DataDAC_In7_CH1"=w496) -> ()  [unwired: 1 in, 1 out]
    n306 = local read "START MAST CH1"() -> (w494:bool)
    n307 = local read "StartAddress8_CH1"() -> (w504:u32)
    n308 = local read "Increment_CH1"() -> (w505:u32)
    n309 = local read "DDS/ARB CH1"() -> (w502:bool)
    n310 = local read "LastAddress_CH1"() -> (w501:u32)
    n311 = local read "Offset_CH1"() -> (w499:u32)
    n312 = call "TableInterface.vi"("Offset"=w499, "LastAddress"=w501, "START"=w494, "DDS/ARB"=w502, "CurrentAddress"=w507, "StopAddress"="StopAddress8_CH1", "StartAddress"=w504, "Increment"=w505) -> ("NextAddress"=w506:u32, "AddressRam"=w503:u32)  [unwired: 1 in, 1 out]
    n313 = xnode ("Memory Write")("Address"=w503) -> ("Data"=w498:fxp<+,14,14>)  [unwired: 1 in, 1 out]
    n314 = local write "LastAddress_CH1"(w506) -> ()
    n315 = node-c288() -> ()  [unwired: 1 out]
  }
  n316 = node-c288(w39) -> ()
  n317 = node-c288(refnum<k21> "IO Module\\iomodclipclock0" ("Source Name")) -> (w32:T2)
  n318 = timed-loop {
    timing: w32 -> [_]
    timing-out: [_] -> w31
    shift-right: [w514] -> _
    shift-left: FALSE -> [w513]
    stop <- _ stop-if-true
    n319 = local read "Trig Selection"() -> (w512:bool)
    n320 = case shown="True" w512 {
      tunnel: [w518 w522] -> w515
      tunnel: w513 -> [_ w521]
      frame False {
        n321 = local read "EN_CH1"() -> (w519:bool)
        n322 = local read "START_CH"() -> (w520:bool)
        n323 = And(x=w520, y=w519) -> (x .and. y?=w518:bool)
      }
      frame True {
        n324 = xnode "FPGA I/O Node"() -> ("PXI_Trig0"=w523)  [unwired: 1 in, 1 out]
        n325 = feedback #4(FALSE ("PXIe_DStarB")) -> (w524:bool)
        n326 = feedback-in #4(w523) -> ()
        n327 = case shown="False" w524 {
          tunnel: w523 -> [w528 _]
          tunnel: [w527 w532] -> w522
          tunnel: w521 -> [w526 w532]
          frame False {
            n328 = case shown="True" w528 {
              tunnel: [w529 w530] -> w527
              tunnel: w526 -> [w529 w531]
              frame False {
              }
              frame True {
                n329 = Not(x=w531) -> (.not. x?=w530:bool)
              }
            }
          }
          frame True {
          }
        }
      }
    }
    n330 = local read "Trig Reset"() -> (w517:bool)
    n331 = Select(t=FALSE, s=w517, f=w515) -> (s? t:f=w514:bool)
    "START MAST CH1" <- w513
  }
  n332 = node-c288(w67) -> ()
  n333 = node-c288(w60) -> ()
  n334 = node-c288(w51) -> ()
  n335 = node-c288(w57) -> ()
  n336 = node-c288(w54) -> ()
  n337 = node-c288(w48) -> ()
  n338 = node-c288(w45) -> ()
  n339 = node-c288(w42) -> ()
  n340 = node-c288(w31) -> ()
  "error out" <- "error in (no error)"
